vi "Draw Markers.vi"(7 "XYGraph in":refnum<vi>, 9 "Marker Options":T3={"Color"=16723218, "pen"={"Width"=2, "Style"=enum."Solid"}, "font"={"Font Name"="Arial", "Size"=16, "Strikeout?"=FALSE, "Italic?"=FALSE, "Underline?"=FALSE, "Outline?"=FALSE, "Shadow?"=FALSE, "Bold?"=FALSE, "FontColor"=0}, "caption"=""}, 10 "Marker":T1={"Type"=enum."vert", "X"=2.0, "Y"=2.0, "X2"=2.0, "Y2"=2.0, "Text"="Drag and click to\nposition a marker"}, 11 "picture":picture) -> (3 "new picture":picture)   [LabVIEW 2015]
doc: "Draw the appropriate line for markers, depending on the type"
uses:
  controls/MarkerOptions.ctl
  controls/MarkerInfo.ctl
  controls/markerType.ctl
  <vilib>/Utility/miscctls.llb/LVPoint32TypeDef.ctl
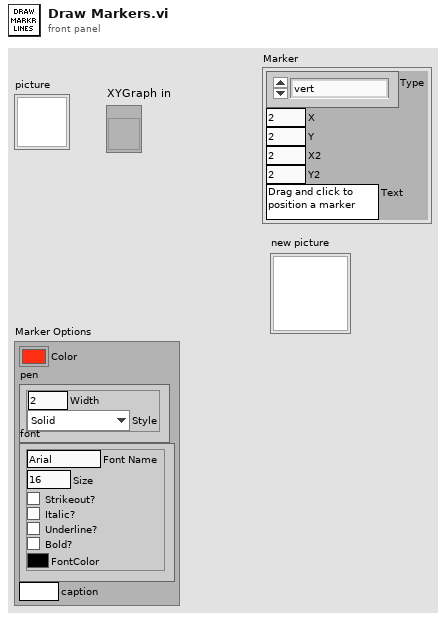
[diagram p1: front panel]
types:
  T1 = typedef "MarkerInfo.ctl" = cluster{"Type":T2, "X":dbl, "Y":dbl, "X2":dbl, "Y2":dbl, "Text":string}
  T2 = typedef "markerType.ctl" = enum16{"point", "arrow", "horiz", "vert", "vert range", "horiz range", "box"}
  T3 = typedef "MarkerOptions.ctl" = cluster{"Color":u32, "pen":cluster{"Width":u16, "Style":enum32{"Solid", "Dash", "Dot", "DashDot", "DashDotDot"}}, "font":cluster{"Font Name":string, "Size":i16, "Strikeout?":bool, "Italic?":bool, "Underline?":bool, "Outline?":bool, "Shadow?":bool, "Bold?":bool, "FontColor":u32}, "caption":string}
  T4 = cluster{"Font Name:":string, "Size":i16, "Strikeout?":bool, "Italic?":bool, "Underline?":bool, "Outline?":bool, "Shadow?":bool, "Bold?":bool}
  T5 = enum16{"User-specified Font", "Application Font", "System Font", "Dialog Font"}
  T6 = typedef "LVPoint32TypeDef.ctl" = cluster{"Horizontal":i32, "Vertical":i32}
  T7 = typedef "LVRectTypeDef.ctl" = cluster{"Left":i16, "Top":i16, "Right":i16, "Bottom":i16}
  T8 = cluster{"Font Name":string, "Size":i16, "Strikeout?":bool, "Italic?":bool, "Underline?":bool, "Outline?":bool, "Shadow?":bool, "Bold?":bool, "FontColor":u32}
  T9 = cluster{"Width":u16, "Style":enum32{"Solid", "Dash", "Dot", "DashDot", "DashDotDot"}}
  T10 = cluster{"left":i16, "top":i16, "right":i16, "bottom":i16}
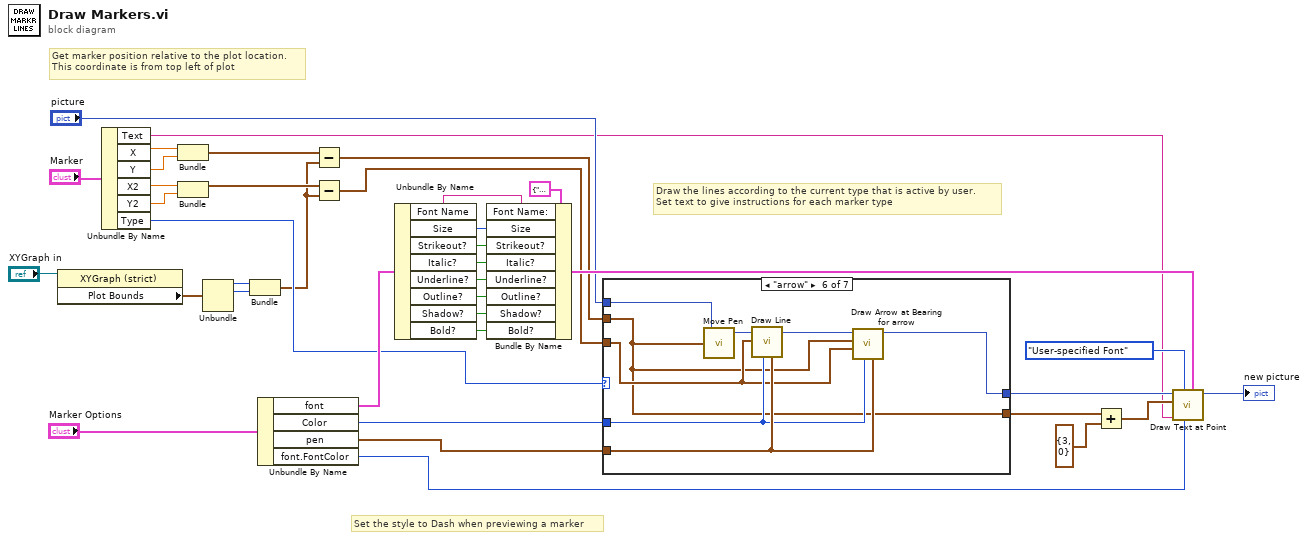
[diagram p0: block diagram]
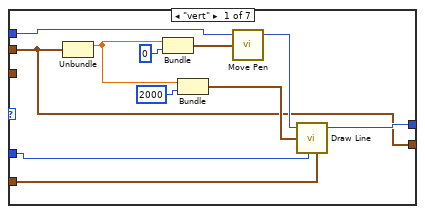
[diagram p2: hidden frame]
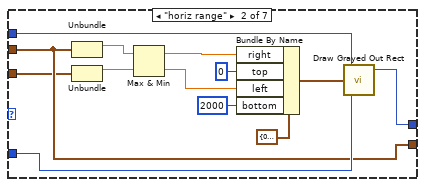
[diagram p3: hidden frame]
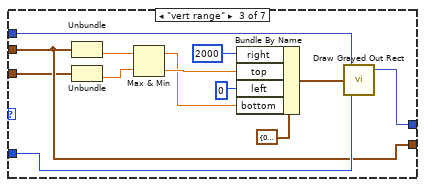
[diagram p4: hidden frame]
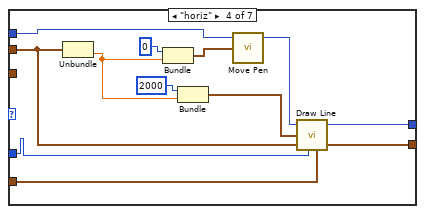
[diagram p5: hidden frame]
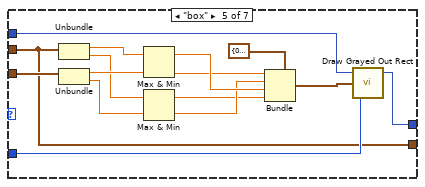
[diagram p6: hidden frame]
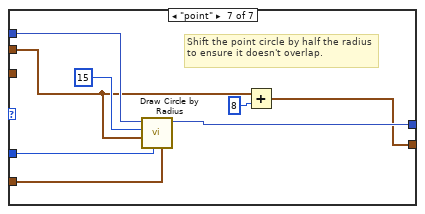
[diagram p7: hidden frame]
diagram:
  # "Get marker position relative to the plot location.\nThis coordinate is from top left of plot"
  # "Set the style to Dash when previewing a marker"
  # "Draw the lines according to the current type that is active by user.\nSet text to give instructions for each marker type"
  n1 = property on="Property Node" class="XYGraph (strict)"(reference="XYGraph in") -> ("Plot Bounds"=w12:T7)  [unwired: 1 in, 2 out]
  n2 = Unbundle By Name("Marker") -> ("Text"=w6:string, "X"=w17:dbl, "Y"=w16:dbl, "X2"=w5:dbl, "Y2"=w4:dbl, "Type"=w7:T2)
  n3 = Bundle("X"=w17, "Y"=w16) -> (w10:cluster{"X":dbl, "Y":dbl})  [unwired: 1 in]
  n4 = Bundle("X2"=w5, "Y2"=w4) -> (w3:cluster{"X2":dbl, "Y2":dbl})  [unwired: 1 in]
  n5 = Unbundle(w12) -> ("Left"=w13:i16, "Top"=w14:i16)  [unwired: 2 out]
  n6 = Bundle("Left"=w13, "Top"=w14) -> (w2:cluster{"Left":i16, "Top":i16})  [unwired: 1 in]
  n7 = Unbundle By Name("Marker Options") -> ("font"=w21:T8, "Color"=w23:u32, "pen"=w8:T9, "font.FontColor"=w34:u32)
  n8 = Subtract(x=w10, y=w2) -> (x-y=w9:cluster{dbl, dbl})
  n9 = Subtract(x=w3, y=w2) -> (x-y=w1:cluster{dbl, dbl})
  n10 = Unbundle By Name(w21) -> ("Font Name"=w32:string, "Size"=w31:i16, "Strikeout?"=w30:bool, "Italic?"=w29:bool, "Underline?"=w28:bool, "Outline?"=w27:bool, "Shadow?"=w26:bool, "Bold?"=w25:bool)
  n11 = Bundle By Name(cluster=T4 {"Font Name:"="", "Size"=12, "Strikeout?"=FALSE, "Italic?"=FALSE, "Underline?"=FALSE, "Outline?"=FALSE, "Shadow?"=FALSE, "Bold?"=FALSE} ("[user-specified font]"), "Font Name:"=w32, "Size"=w31, "Strikeout?"=w30, "Italic?"=w29, "Underline?"=w28, "Outline?"=w27, "Shadow?"=w26, "Bold?"=w25) -> (w24:T4)
  n12 = case shown="\"arrow\"" w7 {
    tunnel: w9 -> [w39 w60 w73 w79 w87 w102 w112]
    tunnel: [w47 w62 w75 w85 w99 w106 w117] -> w36
    tunnel: "picture" -> [w42 w54 w69 w76 w101 w108 w113]
    tunnel: w23 -> [w41 w61 w74 w78 w100 w104 w116]
    tunnel: w8 -> [w40 _ _ w77 _ w105 w114]
    tunnel: [w39 w60 w73 w79 w87 w102 w110] -> w22
    tunnel: w1 -> [_ w55 w70 _ w96 w103 _]
    frame "vert" {
      n13 = Unbundle(w39) -> (w49:dbl)  [unwired: 1 out]
      n14 = Bundle(w49, "top"=i16 0) -> (w43:cluster{dbl, "top":i16})  [unwired: 1 in]
      n15 = Bundle(w49, "top"=i16 2000) -> (w48:cluster{dbl, "top":i16})  [unwired: 1 in]
      n16 = call <vilib>:"Move Pen.vi"("new position"=w43, "picture"=w42) -> ("new picture"=w46:picture)  [unwired: 3 in]
      n17 = call <vilib>:"Draw Line.vi"("picture"=w46, "end point"=w48, "color(black)"=w41, "pen"=w40) -> ("new picture"=w47:picture)  [unwired: 5 in]
    }
    frame "horiz range" {
      n18 = Unbundle(w60) -> (w53:dbl)  [unwired: 1 out]
      n19 = Unbundle(w55) -> (w52:dbl)  [unwired: 1 out]
      n20 = Max & Min(x=w53, y=w52) -> (max(x,y)=w50:dbl, min(x,y)=w51:dbl)
      n21 = Bundle By Name(cluster=T10 {"left"=0, "top"=0, "right"=0, "bottom"=0} ("rect"), "right"=w50, "top"=i16 0, "left"=w51, "bottom"=i16 2000) -> (w58:T10)
      n22 = call <vilib>:"Draw Grayed Out Rect.vi"("color(black)"=w61, "rect"=w58, "picture"=w54) -> ("new picture"=w62:picture)  [unwired: 2 in]
    }
    frame "vert range" {
      n23 = Unbundle(w73) -> (w68:dbl)  [unwired: 1 out]
      n24 = Unbundle(w70) -> (w67:dbl)  [unwired: 1 out]
      n25 = Max & Min(x=w68, y=w67) -> (max(x,y)=w63:dbl, min(x,y)=w64:dbl)
      n26 = Bundle By Name(cluster=T10 {"left"=0, "top"=0, "right"=0, "bottom"=0} ("rect"), "right"=i16 2000 ("top"), "top"=w64, "left"=i16 0 ("bottom"), "bottom"=w63) -> (w71:T10)
      n27 = call <vilib>:"Draw Grayed Out Rect.vi"("color(black)"=w74, "rect"=w71, "picture"=w69) -> ("new picture"=w75:picture)  [unwired: 2 in]
    }
    frame "horiz" {
      n28 = Unbundle(w79) -> (w81:dbl)  [unwired: 1 out]
      n29 = Bundle("top"=i16 0, w81) -> (w83:cluster{"top":i16, dbl})  [unwired: 1 in]
      n30 = Bundle("top"=i16 2000, w81) -> (w86:cluster{"top":i16, dbl})  [unwired: 1 in]
      n31 = call <vilib>:"Move Pen.vi"("new position"=w83, "picture"=w76) -> ("new picture"=w84:picture)  [unwired: 3 in]
      n32 = call <vilib>:"Draw Line.vi"("picture"=w84, "end point"=w86, "color(black)"=w78, "pen"=w77) -> ("new picture"=w85:picture)  [unwired: 5 in]
    }
    frame "box" {
      n33 = Unbundle(w87) -> (w95:dbl, w91:dbl)
      n34 = Unbundle(w96) -> (w94:dbl, w90:dbl)
      n35 = Max & Min(x=w95, y=w94) -> (max(x,y)=w93:dbl, min(x,y)=w92:dbl)
      n36 = Max & Min(x=w91, y=w90) -> (max(x,y)=w88:dbl, min(x,y)=w89:dbl)
      n37 = Bundle(cluster=T10 {"left"=0, "top"=0, "right"=0, "bottom"=0} ("rect"), "left"=w92, "top"=w89, "right"=w93, "bottom"=w88) -> (w98:T10)
      n38 = call <vilib>:"Draw Grayed Out Rect.vi"("color(black)"=w100, "rect"=w98, "picture"=w101) -> ("new picture"=w99:picture)  [unwired: 2 in]
    }
    frame "arrow" {
      n39 = call <vilib>:"Move Pen.vi"("new position"=w102, "picture"=w108) -> ("new picture"=w109:picture)  [unwired: 3 in]
      n40 = call <vilib>:"Draw Line.vi"("picture"=w109, "end point"=w103, "color(black)"=w104, "pen"=w105) -> ("new picture"=w107:picture)  [unwired: 5 in]
      n41 = call "Draw Arrow at Bearing for arrow.vi"("pen"=w105, "color(black)"=w104, "P2"=w103, "P1"=w102, "new picture in"=w107) -> ("new picture out"=w106:picture)  [unwired: 6 in]
    }
    frame "point" {
      # "Shift the point circle by half the radius to ensure it doesn't overlap."
      n42 = call <vilib>:"Draw Circle by Radius.vi"("pen"=w114, "color(black)"=w116, "pixel center"=w112, "radius"=i16 15, "picture"=w113) -> ("new picture"=w117:picture)  [unwired: 6 in]
      n43 = Add(x=w112, y=8 ("Horizontal")) -> (x+y=w110:cluster{dbl, dbl})
    }
  }
  n44 = Add(x=w22, y=T6 {"Horizontal"=3, "Vertical"=0}) -> (x+y=w37:cluster{dbl, dbl})
  n45 = call <vilib>:"Draw Text at Point.vi"("[user-specified font]"=w24, "text color(black)"=w34, "desired font(Application)"=T5."User-specified Font", "text"=w6, "origin"=w37, "picture"=w36) -> ("new picture"=→"new picture":picture)  [unwired: 4 in, 1 out]
